vi "DFD Build Filter from Cascaded Coef.vi"(6 "fs [Hz]":dbl=1.0 format="%.2f", 8 "error in (no error)":errorcluster, 10 "IIR Filter Cluster":T1) -> (0 "error out":errorcluster, 3 "filter out":T2={"mSRate_Fs"=1.0, "mSRate_Version"="2.0", "mSRate_Comments"="", "mSRate_OrgCoef"={"type"=enum."Undefined", "gain"=1.0, "coef a (k)"=[], "coef b (v)"=[]}, "mSRate_CurCoef"={"type"=enum."Undefined", "gain"=1.0, "coef a (k)"=[], "coef b (v)"=[]}, "mSRate_Quantized?"=FALSE, "mSRate_QCoef"={"type"=enum."Undefined", "gain"=1.0, "coef a (k)"=[], "coef b (v)"=[]}, "mSRate_QSettings"=[], "mSRate_Order"=0, "mSRate_Scaling"={"mSRate_ScaleByPowerOf2?"=FALSE, "mSRate_ScaleType"=enum."No Norm"}} {"mSRate_QSettings"."source" items=["Coef a/k"=0, "Coef b/v"=7, "Input"=1, "Output"=2, "Multiplicand"=3, "Product"=4, "Sum"=5, "Delay"=6, "Gain"=8]})   [LabVIEW 2017, in "NI_DigFilterLicensed.lvlib"]
doc: "Converts the <B>IIR Filter Cluster</B> output of the Advanced IIR Filtering VIs into a filter."
uses:
  <vilib>/addons/Digital Filter Design/NI_DigFilterLicensed.lvlib
  <vilib>/addons/Digital Filter Design/_Objects.llb/DFD Filter Obj.ctl
  <vilib>/addons/Digital Filter Design/_Objects.llb/DFD Filter Coef.ctl
  <vilib>/addons/Digital Filter Design/_Objects.llb/DFD Filter Structure Type Selector.ctl
  <vilib>/addons/Digital Filter Design/_Objects.llb/dfd_Internal Quantization Settings.ctl
  <vilib>/addons/Digital Filter Design/_Objects.llb/dfd_Internal Quantization Srcs.ctl
  <vilib>/addons/Digital Filter Design/_Objects.llb/DFD Coef Norm Type.ctl
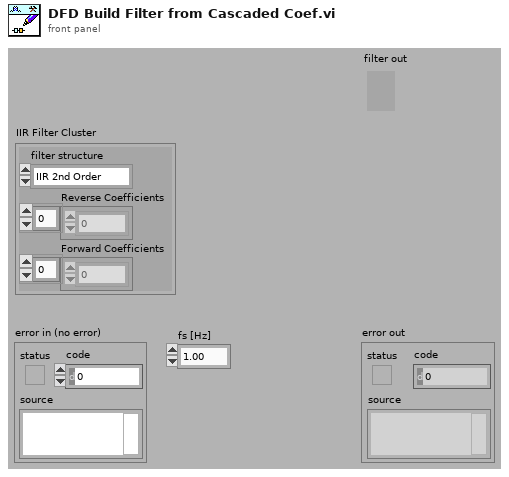
[diagram p1: front panel]
types:
  T1 = cluster{"filter structure":enum32{"IIR 2nd Order", "IIR 4th Order"}, "Reverse Coefficients":dbl[], "Forward Coefficients":dbl[]}
  T2 = typedef "NI_DigFilterLicensed.lvlib/DFD Filter Obj.ctl" = cluster{"mSRate_Fs":dbl, "mSRate_Version":string, "mSRate_Comments":string, "mSRate_OrgCoef":T3, "mSRate_CurCoef":T3, "mSRate_Quantized?":bool, "mSRate_QCoef":T3, "mSRate_QSettings":T5[], "mSRate_Order":i32, "mSRate_Scaling":cluster{"mSRate_ScaleByPowerOf2?":bool, "mSRate_ScaleType":T7}}
  T3 = typedef "NI_DigFilterLicensed.lvlib/DFD Filter Coef.ctl" = cluster{"type":T4, "gain":dbl, "coef a (k)":dbl[], "coef b (v)":dbl[]}
  T4 = typedef "NI_DigFilterLicensed.lvlib/DFD Filter Structure Type Selector.ctl" = enum16{"Undefined", "FIR Direct Form", "FIR Direct Form Transposed", "FIR Symmetric", "FIR Antisymmetric", "IIR Direct Form I", "IIR Direct Form I Transposed", "IIR Direct Form II", "IIR Direct Form II Transposed", "IIR Cascaded Second Order Sections Form I", "IIR Cascaded Second Order Sections Form I Transposed", "IIR Cascaded Second Order Sections Form II", "IIR Cascaded Second Order Sections Form II Transposed", "Lattice Allpass (basic sections)", "Lattice Allpass (one multiplier sections)", "Lattice Allpass (normalized sections)", "Lattice AR (basic sections)", "Lattice AR (one multiplier sections)", "Lattice AR (normalized sections)", "Lattice MA (minimum phase)", "Lattice MA (maximum phase)", "Lattice ARMA (basic sections)", "Lattice ARMA (one multiplier sections)", "Lattice ARMA (normalized sections)"}
  T5 = typedef "NI_DigFilterLicensed.lvlib/dfd_Internal Quantization Settings.ctl" = cluster{"source":T6, "wl":i16, "iwl":i16, "overflow mode":enum16{"Saturation", "Wrap"}, "rounding mode":enum16{"Nearest", "Truncation"}, "signed?":bool}
  T6 = typedef "NI_DigFilterLicensed.lvlib/dfd_Internal Quantization Srcs.ctl" = u16
  T7 = typedef "NI_DigFilterLicensed.lvlib/DFD Coef Norm Type.ctl" = enum16{"No Norm", "Time Domain 1-Norm", "Time Domain 2-Norm", "Time Domain Inf-Norm"}
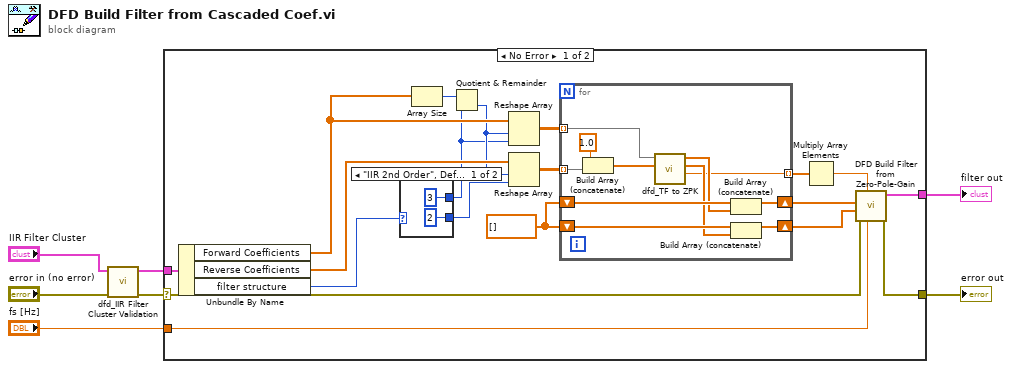
[diagram p0: block diagram]
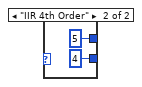
[diagram p2: hidden frame]
diagram:
  n1 = call <vilib>:"dfd_IIR Filter Cluster Validation.vi"("error in (no error)"="error in (no error)", "IIR Filter Cluster"="IIR Filter Cluster") -> ("error out"=w5:errorcluster, "dup IIR Filter Cluster"=w3:T1)  [unwired: 8 out]
  n2 = case shown="No Error" w5 {
    selector: w5 -> [w16 w42]
    tunnel: w3 -> [w24 _]
    tunnel: [w17 w42] -> w6
    tunnel: [w18 _] -> w7
    tunnel: "fs [Hz]" -> [w8 _]
    frame No Error {
      w22 = cdb[] []
      n3 = Unbundle By Name(w24) -> ("Forward Coefficients"=w26:dbl[], "Reverse Coefficients"=w25:dbl[], "filter structure"=w11:enum32{"IIR 2nd Order", "IIR 4th Order"})
      n4 = case shown="\"IIR 2nd Order\", Default" w11 {
        tunnel: [3 ("y") 5 ("y")] -> w9
        tunnel: [2 ("y") 4 ("y")] -> w10
        frame "IIR 2nd Order", Default {
        }
        frame "IIR 4th Order" {
        }
      }
      n5 = Array Size(array=w26) -> (size(s)=w23:i32)
      n6 = Quotient & Remainder(x=w23, y=w9) -> (floor(x/y)=w21:i32)  [unwired: 1 out]
      n7 = Reshape Array(w26, w21, w9) -> (w19:dbl[][])
      n8 = Reshape Array(w25, w21, w10) -> (w20:dbl[][])
      n9 = for {
        shift-right: [w37] -> w14
        shift-left: w22 -> [w40]
        shift-right: [w38] -> w15
        shift-left: w22 -> [w41]
        tunnel: w20 -> [w36] mode=indexing
        tunnel: w19 -> [w35] mode=indexing
        tunnel: [w31] -> w13 mode=indexing
        n10 = Build Array (concatenate)(1.0, w36) -> (w34:dbl[])
        n11 = call <vilib>:"dfd_TF to ZPK.vi"("denominator"=w34, "numerator"=w35) -> ("gain"=w31:dbl, "poles"=w32:cdb[], "zeros"=w33:cdb[])  [unwired: 7 out]
        n12 = Build Array (concatenate)(w41, w33) -> (w38:cdb[])
        n13 = Build Array (concatenate)(w40, w32) -> (w37:cdb[])
      }
      n14 = Multiply Array Elements(1:w13) -> (0:w12:dbl)
      n15 = call <vilib>:"DFD Build Filter from Zero-Pole-Gain.vi"("fs [Hz]"=w8, "gain"=w12, "error in (no error)"=w16, "poles"=w14, "zeroes"=w15) -> ("error out"=w17:errorcluster, "filter out"=w18:T2)  [unwired: 5 out]
    }
    frame Error {
    }
  }
  "filter out" <- w7
  "error out" <- w6
